vi "Configure Timing's.vi"(7 "Data Cluster In":T1, 8 "error in (no error)":errorcluster, 11 "Configuration Data":variant) -> (0 "error out":errorcluster, 5 "Data Cluster Out":T1)   [LabVIEW 2021, in "RT-AutoSequence.lvlib"]
uses:
  RT-AutoSequence.lvlib
  Module Data--cluster.ctl
  TCP Engine/Controls/TCP Engine I&O  Interupt Cluster.ctl
  TCP Engine/TCP Engine.lvlib
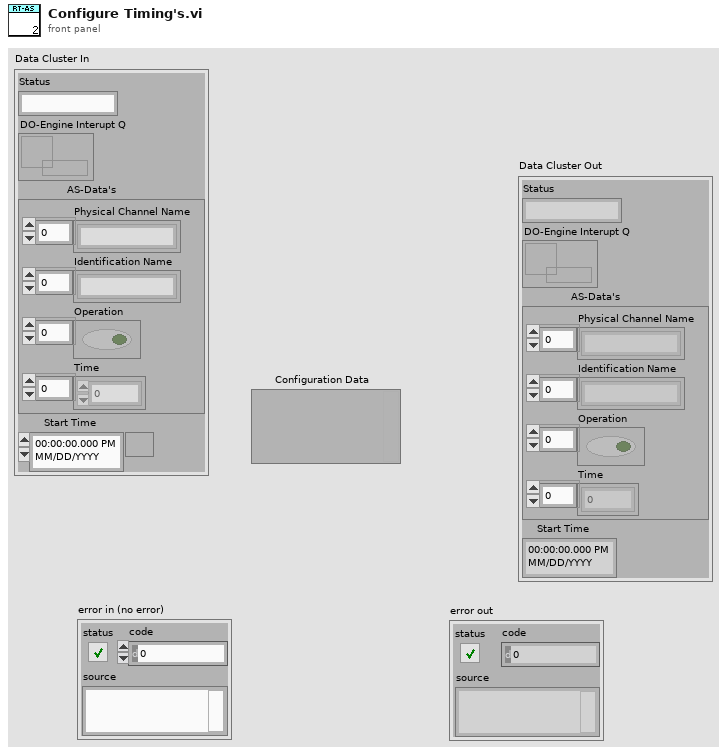
[diagram p1: front panel]
types:
  T1 = typedef "RT-AutoSequence.lvlib/Module Data--cluster.ctl" = cluster{"Status":string, "DO-Engine Interupt Q":refnum<queue>, "AS-Data's":cluster{"Physical Channel Name":string[], "Identification Name":string[], "Operation":bool[], "Time":dbl[]}, "Start Time":timestamp}
  T2 = cluster{"Physical Channel Name":string, "Identification Name":string, "Operation":bool, "Time":dbl}[]
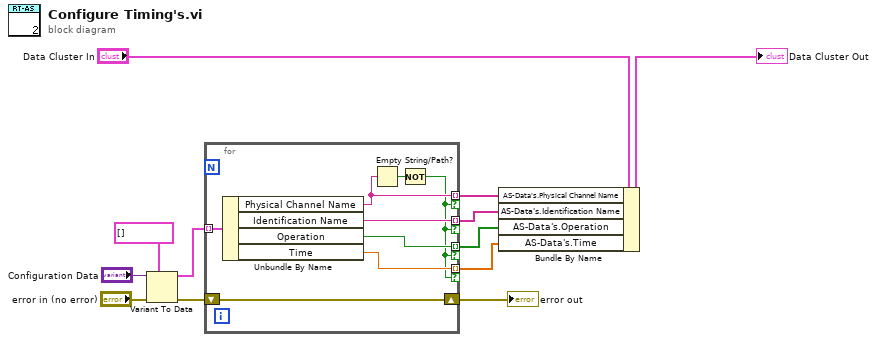
[diagram p0: block diagram]
diagram:
  n1 = Variant To Data(error in="error in (no error)", type=T2 [], Variant="Configuration Data") -> (data=w12:T2, error out=w11:errorcluster)
  n2 = for {
    tunnel: w12 -> [w19] mode=indexing
    shift-right: [w20] -> w8
    shift-left: w11 -> [w20]
    tunnel: [w18] -> w3 mode=indexing if=w13
    tunnel: [w17] -> w2 mode=indexing if=w13
    tunnel: [w16] -> w1 mode=indexing if=w13
    tunnel: [w14] -> w4 mode=indexing if=w13
    n3 = Unbundle By Name(w19) -> ("Physical Channel Name"=w14:string, "Identification Name"=w18:string, "Operation"=w17:bool, "Time"=w16:dbl)
    n4 = Empty String/Path?(string/path=w14) -> (empty?=w15:bool)
    n5 = Not(x=w15) -> (.not. x?=w13:bool)
  }
  "error out" <- w8
  n6 = Bundle By Name(cluster="Data Cluster In", "AS-Data's.Physical Channel Name"=w4, "AS-Data's.Identification Name"=w3, "AS-Data's.Operation"=w2, "AS-Data's.Time"=w1) -> (→"Data Cluster Out":T1)
